vi "Untitled 2.vi"() -> ()   [LabVIEW 2015]
panel:
  in  "stop":bool
  out "Boolean 2":bool
  in  "Boolean":bool
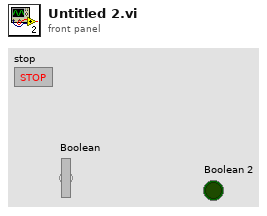
[diagram p1: front panel]
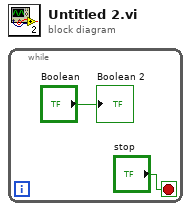
[diagram p0: block diagram]
diagram:
  n1 = while {
    stop <- "stop" stop-if-true
    "Boolean 2" <- "Boolean"
  }
